vi "OFDM_Demodulation.vi"(9 "sampling period":dbl format="%#_13g", 10 "Frequency channel estimation":cdb[](array[numeric]) format="%.2f", 11 "Input sequence":cdb[](array[numeric])) -> (2 "FFT":dbl[](graph), 3 "Output sequence":cdb[](array[numeric]))   [LabVIEW 2022 SP3]
uses:
  <vilib>/Analysis/2dsp.llb/Complex FFT.vi
  <vilib>/Analysis/baseanly.llb/Mean (CDB).vi
  <vilib>/Analysis/NI_AALPro.lvlib
  <vilib>/Analysis/NI_AALBase.lvlib
panel:
  out "size(s) 2":i32
  out "x/y":cdb[](array[numeric])
  out "Waveform Graph":dbl[](graph)
  out "size(s)":i32
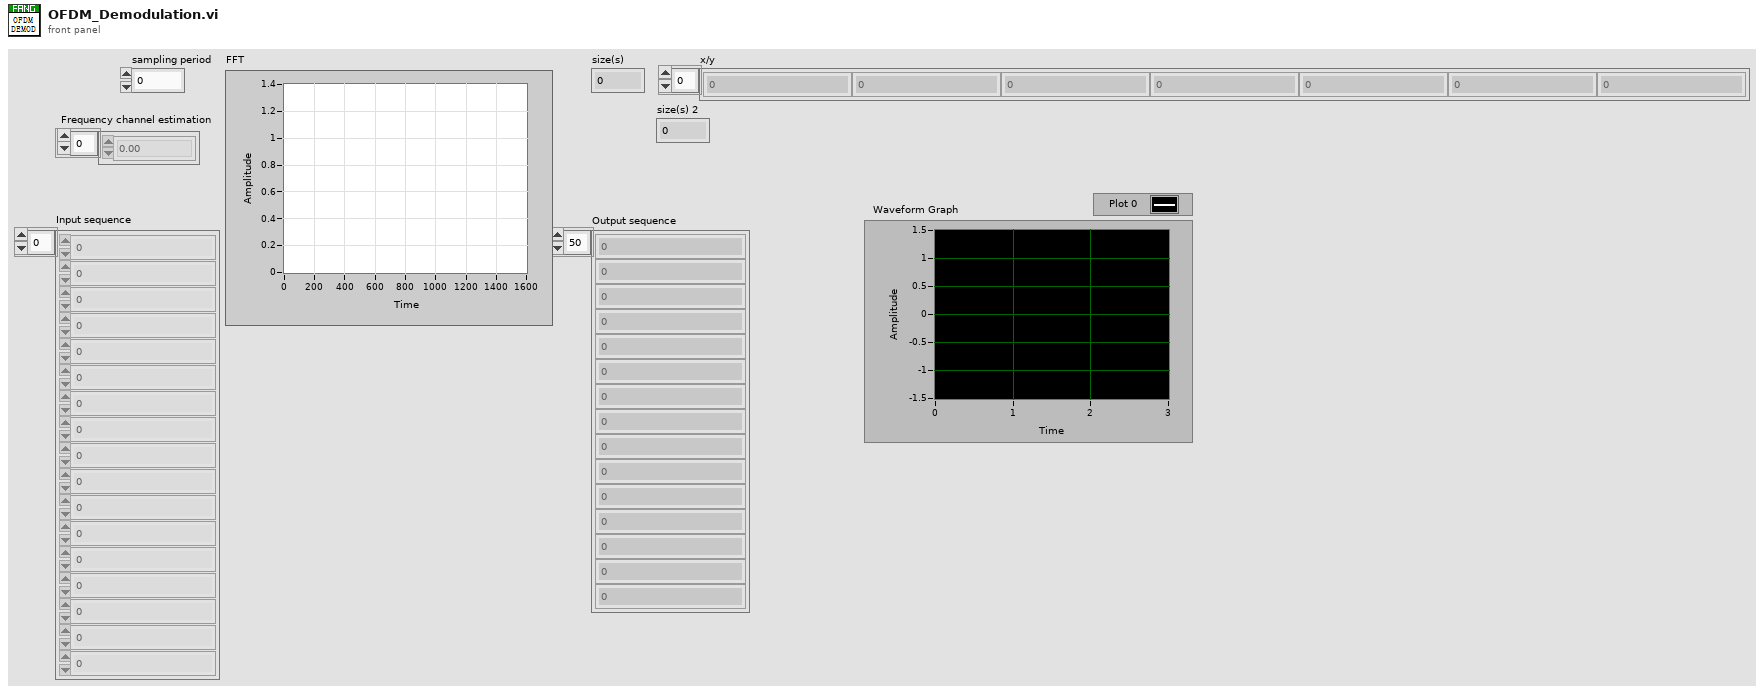
[diagram p1: front panel]
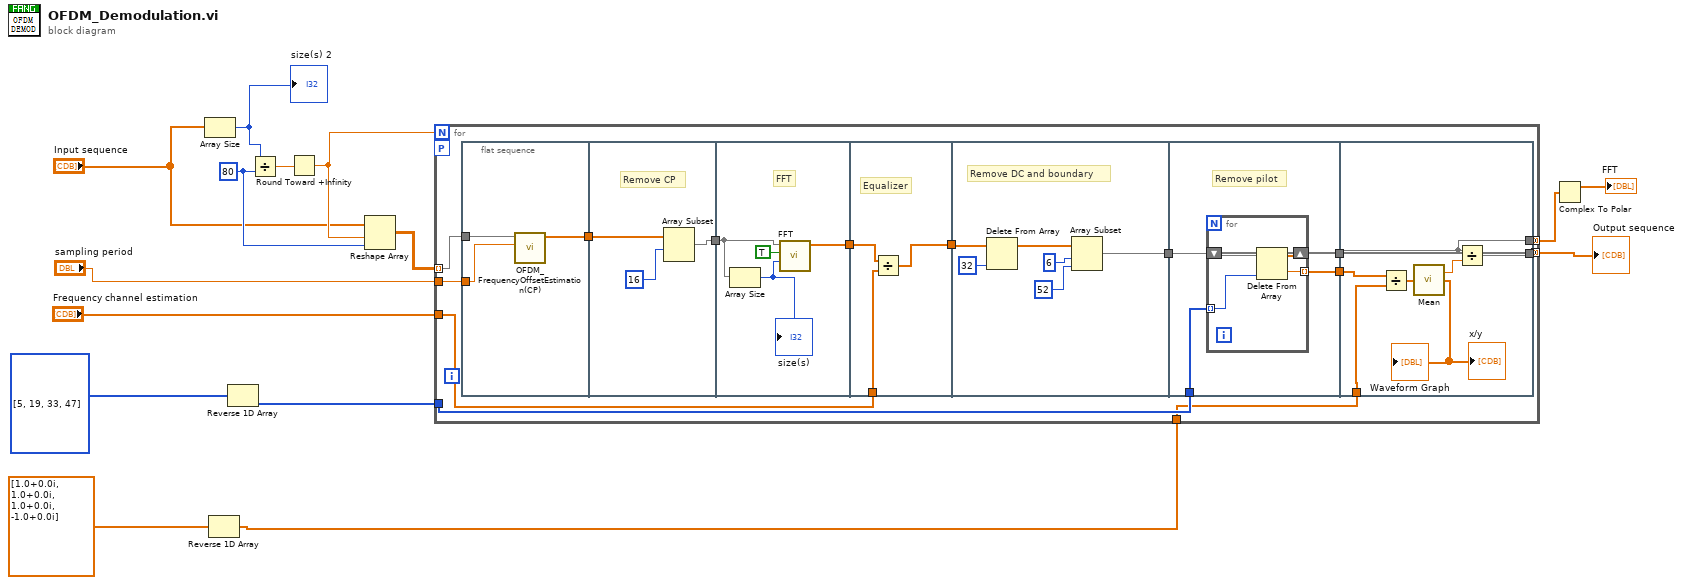
[diagram p0: block diagram]
diagram:
  w11 = 80 ("y")
  n1 = Array Size(array="Input sequence") -> (size(s)=w15:i32)
  "size(s) 2" <- w15
  n2 = Reverse 1D Array(array=cdb[] [1.0+0.0i, 1.0+0.0i, 1.0+0.0i, -1.0+0.0i]) -> (reversed array=w5:cdb[])
  n3 = Reverse 1D Array(array=i32[] [5, 19, 33, 47]) -> (reversed array=w9:i32[])
  n4 = Divide(x=w15, y=w11) -> (x/y=w14:dbl)
  n5 = Round Toward +Infinity(x=w14) -> (ceil(x): smallest int >= x=w12:dbl)
  n6 = Reshape Array("Input sequence", w12, w11) -> (w13:cdb[][])
  n7 = for {
    N: w12 -> [_]
    tunnel: w13 -> [w27] mode=indexing
    tunnel: w9 -> [w28]
    tunnel: [w22] -> w2 mode=concatenating
    tunnel: "Frequency channel estimation" -> [w24]
    tunnel: w5 -> [w19]
    workers-P: _ -> [_]
    tunnel: "sampling period" -> [w17]
    tunnel: [w16] -> w1 mode=concatenating
    n8 = flat-sequence {
      tunnel: w27 -> [w32]
      tunnel: [w30] -> w18
      tunnel: w17 -> [w31]
      tunnel: [w33] -> w25
      tunnel: w18 -> [w35]
      tunnel: [w36] -> w26
      tunnel: w25 -> [w37]
      tunnel: w26 -> [w41]
      tunnel: w24 -> [w42]
      tunnel: [w40] -> w23
      tunnel: [w43] -> w29
      tunnel: w23 -> [w46]
      tunnel: w29 -> [w50]
      tunnel: w28 -> [w52]
      tunnel: [w49] -> w21
      tunnel: [w51] -> w20
      tunnel: [w60] -> w22
      tunnel: w21 -> [w57]
      tunnel: w20 -> [w59]
      tunnel: w19 -> [w62]
      tunnel: [w57] -> w16
      frame #0 {
        n9 = call "OFDM_FrequencyOffsetEstimation(CP).vi"("sampling period"=w31, "input OFDM symbol"=w32) -> ("output OFDM symbol"=w30:cdb[])  [unwired: 9 in]
      }
      frame #1 {
        # "Remove CP"
        n10 = Array Subset(array=w35, index=16) -> (w33:cdb[])  [unwired: 1 in]
      }
      frame #2 {
        # "FFT"
        n11 = Array Size(array=w37) -> (size(s)=w38:i32)
        "size(s)" <- w38
        n12 = call-poly <vilib>:"FFT.vi"("FFT size"=w38, "shift?"=TRUE, "X"=w37) -> ("FFT {X}"=w36:cdb[])  [unwired: 7 in, 1 out]
      }
      frame #3 {
        # "Equalizer"
        n13 = Divide(x=w41, y=w42) -> (x/y=w40:cdb[])
      }
      frame #4 {
        # "Remove DC and boundary"
        n14 = Delete From Array(array=w46, index=32) -> (array with subset deleted=w44:cdb[])  [unwired: 1 in, 1 out]
        n15 = Array Subset(array=w44, index=6, length=52) -> (w43:cdb[])
      }
      frame #5 {
        # "Remove pilot"
        n16 = for {
          shift-right: [w56] -> w49
          shift-left: w50 -> [w55]
          tunnel: w52 -> [w54] mode=indexing
          tunnel: [w53] -> w51 mode=indexing
          n17 = Delete From Array(array=w55, index=w54) -> (deleted portion=w53:cdb, array with subset deleted=w56:cdb[])  [unwired: 1 in]
        }
      }
      frame #6 {
        n18 = Divide(x=w59, y=w62) -> (x/y=w58:cdb[])
        "Waveform Graph" <- w58
        "x/y" <- w58
        n19 = call-poly <vilib>:"Mean.vi"("X"=w58) -> ("mean"=w61:cdb)  [unwired: 1 out]
        n20 = Divide(x=w57, y=w61) -> (x/y=w60:cdb[])
      }
    }
  }
  "Output sequence" <- w2
  n21 = Complex To Polar(r * e^(i*theta)=w1) -> (r=→"FFT":dbl[])  [unwired: 1 out]
